vi "guangzi_16.vi"() -> ()   [LabVIEW 2016]
uses:
  <vilib>/Utility/file.llb/Write To Spreadsheet File (DBL).vi
panel:
  in  "采集开关":bool
  out "切片图":u32[](graph)
  in  "切片值":i32
  in  "选项卡控件":T1(tab)
  in  "对数":bool
  out "MCS8Dat Error":i32
  out "CHN Status":T2 {"Dummy" format="%.2f"; "Starts" format="%.2f"; "Sweeps" format="%.2f"; "Roirate" format="%.2f"; "RoiSum" format="%.2f"; "TotalSum" format="%.2f"; "Fifo full" format="%.2f"; "Runtime" format="%.2f"}
  out "Data":u32[](graph)
  out "Settings":T3 {"dummy3" format="%.2f"; "dummy2" format="%.2f"; "bitshift" format="%.0x"; "Active" format="%.0x"; "Offset" format="%.0x"; "Param" format="%.0x"; "dummy1" format="%.2f"; "Roipreset" format="%.2f"; "cftfak" format="%.0x"}
  out "通道数":i32
  out "Data 9":dbl[](graph)
  out "Data 2":u32[](graph)
  out "MCS8Dat Error 2":i32
  out "Settings 2":T3 {"dummy3" format="%.2f"; "dummy2" format="%.2f"; "bitshift" format="%.0x"; "Active" format="%.0x"; "Offset" format="%.0x"; "Param" format="%.0x"; "dummy1" format="%.2f"; "Roipreset" format="%.2f"; "cftfak" format="%.0x"}
  out "CHN Status 2":T2 {"Dummy" format="%.2f"; "Starts" format="%.2f"; "Sweeps" format="%.2f"; "Roirate" format="%.2f"; "RoiSum" format="%.2f"; "TotalSum" format="%.2f"; "Fifo full" format="%.2f"; "Runtime" format="%.2f"}
  out "通道数 2":i32
  in  "对数 2":bool
  out "Data10":dbl[](graph)
  out "Data 3":u32[](graph)
  out "MCS8Dat Error 3":i32
  out "Settings 3":T3 {"dummy3" format="%.2f"; "dummy2" format="%.2f"; "bitshift" format="%.0x"; "Active" format="%.0x"; "Offset" format="%.0x"; "Param" format="%.0x"; "dummy1" format="%.2f"; "Roipreset" format="%.2f"; "cftfak" format="%.0x"}
  out "CHN Status 3":T2 {"Dummy" format="%.2f"; "Starts" format="%.2f"; "Sweeps" format="%.2f"; "Roirate" format="%.2f"; "RoiSum" format="%.2f"; "TotalSum" format="%.2f"; "Fifo full" format="%.2f"; "Runtime" format="%.2f"}
  out "通道数 3":i32
  in  "对数 3":bool
  out "Data10 2":dbl[](graph)
  out "Data 4":u32[](graph)
  out "MCS8Dat Error 4":i32
  out "Settings 4":T3 {"dummy3" format="%.2f"; "dummy2" format="%.2f"; "bitshift" format="%.0x"; "Active" format="%.0x"; "Offset" format="%.0x"; "Param" format="%.0x"; "dummy1" format="%.2f"; "Roipreset" format="%.2f"; "cftfak" format="%.0x"}
  out "CHN Status 4":T2 {"Dummy" format="%.2f"; "Starts" format="%.2f"; "Sweeps" format="%.2f"; "Roirate" format="%.2f"; "RoiSum" format="%.2f"; "TotalSum" format="%.2f"; "Fifo full" format="%.2f"; "Runtime" format="%.2f"}
  out "通道数 4":i32
  in  "对数 4":bool
  out "Data10 3":dbl[](graph)
  out "Data 5":u32[](graph)
  out "MCS8Dat Error 5":i32
  out "Settings 5":T3 {"dummy3" format="%.2f"; "dummy2" format="%.2f"; "bitshift" format="%.0x"; "Active" format="%.0x"; "Offset" format="%.0x"; "Param" format="%.0x"; "dummy1" format="%.2f"; "Roipreset" format="%.2f"; "cftfak" format="%.0x"}
  out "CHN Status 5":T2 {"Dummy" format="%.2f"; "Starts" format="%.2f"; "Sweeps" format="%.2f"; "Roirate" format="%.2f"; "RoiSum" format="%.2f"; "TotalSum" format="%.2f"; "Fifo full" format="%.2f"; "Runtime" format="%.2f"}
  out "通道数 5":i32
  in  "对数 5":bool
  out "Data10 4":dbl[](graph)
  out "Data 6":u32[](graph)
  out "MCS8Dat Error 6":i32
  out "Settings 6":T3 {"dummy3" format="%.2f"; "dummy2" format="%.2f"; "bitshift" format="%.0x"; "Active" format="%.0x"; "Offset" format="%.0x"; "Param" format="%.0x"; "dummy1" format="%.2f"; "Roipreset" format="%.2f"; "cftfak" format="%.0x"}
  out "CHN Status 6":T2 {"Dummy" format="%.2f"; "Starts" format="%.2f"; "Sweeps" format="%.2f"; "Roirate" format="%.2f"; "RoiSum" format="%.2f"; "TotalSum" format="%.2f"; "Fifo full" format="%.2f"; "Runtime" format="%.2f"}
  out "通道数 6":i32
  in  "对数 6":bool
  out "Data10 5":dbl[](graph)
  out "Data 7":u32[](graph)
  out "MCS8Dat Error 7":i32
  out "Settings 7":T3 {"dummy3" format="%.2f"; "dummy2" format="%.2f"; "bitshift" format="%.0x"; "Active" format="%.0x"; "Offset" format="%.0x"; "Param" format="%.0x"; "dummy1" format="%.2f"; "Roipreset" format="%.2f"; "cftfak" format="%.0x"}
  out "CHN Status 7":T2 {"Dummy" format="%.2f"; "Starts" format="%.2f"; "Sweeps" format="%.2f"; "Roirate" format="%.2f"; "RoiSum" format="%.2f"; "TotalSum" format="%.2f"; "Fifo full" format="%.2f"; "Runtime" format="%.2f"}
  out "通道数 7":i32
  in  "对数 7":bool
  out "Data10 6":dbl[](graph)
  out "Data 8":u32[](graph)
  out "MCS8Dat Error 8":i32
  out "Settings 8":T3 {"dummy3" format="%.2f"; "dummy2" format="%.2f"; "bitshift" format="%.0x"; "Active" format="%.0x"; "Offset" format="%.0x"; "Param" format="%.0x"; "dummy1" format="%.2f"; "Roipreset" format="%.2f"; "cftfak" format="%.0x"}
  out "CHN Status 8":T2 {"Dummy" format="%.2f"; "Starts" format="%.2f"; "Sweeps" format="%.2f"; "Roirate" format="%.2f"; "RoiSum" format="%.2f"; "TotalSum" format="%.2f"; "Fifo full" format="%.2f"; "Runtime" format="%.2f"}
  out "通道数 8":i32
  in  "对数 8":bool
  out "Data10 7":dbl[](graph)
  out "Data9":u32[](graph)
  out "MCS8Dat Error 9":i32
  out "Settings 9":T3 {"dummy3" format="%.2f"; "dummy2" format="%.2f"; "bitshift" format="%.0x"; "Active" format="%.0x"; "Offset" format="%.0x"; "Param" format="%.0x"; "dummy1" format="%.2f"; "Roipreset" format="%.2f"; "cftfak" format="%.0x"}
  out "CHN Status 9":T2 {"Dummy" format="%.2f"; "Starts" format="%.2f"; "Sweeps" format="%.2f"; "Roirate" format="%.2f"; "RoiSum" format="%.2f"; "TotalSum" format="%.2f"; "Fifo full" format="%.2f"; "Runtime" format="%.2f"}
  out "通道数 9":i32
  in  "对数 9":bool
  out "Data108":dbl[](graph)
  in  "对数 10":bool
  out "通道数 10":i32
  out "CHN Status 10":T2 {"Dummy" format="%.2f"; "Starts" format="%.2f"; "Sweeps" format="%.2f"; "Roirate" format="%.2f"; "RoiSum" format="%.2f"; "TotalSum" format="%.2f"; "Fifo full" format="%.2f"; "Runtime" format="%.2f"}
  out "Settings 10":T3 {"dummy3" format="%.2f"; "dummy2" format="%.2f"; "bitshift" format="%.0x"; "Active" format="%.0x"; "Offset" format="%.0x"; "Param" format="%.0x"; "dummy1" format="%.2f"; "Roipreset" format="%.2f"; "cftfak" format="%.0x"}
  out "MCS8Dat Error 10":i32
  out "Data10 8":u32[](graph)
  out "Data10 9":dbl[](graph)
  in  "对数 11":bool
  out "通道数 11":i32
  out "CHN Status 11":T2 {"Dummy" format="%.2f"; "Starts" format="%.2f"; "Sweeps" format="%.2f"; "Roirate" format="%.2f"; "RoiSum" format="%.2f"; "TotalSum" format="%.2f"; "Fifo full" format="%.2f"; "Runtime" format="%.2f"}
  out "Settings 11":T3 {"dummy3" format="%.2f"; "dummy2" format="%.2f"; "bitshift" format="%.0x"; "Active" format="%.0x"; "Offset" format="%.0x"; "Param" format="%.0x"; "dummy1" format="%.2f"; "Roipreset" format="%.2f"; "cftfak" format="%.0x"}
  out "MCS8Dat Error 11":i32
  out "Data11":u32[](graph)
  out "Data10 10":dbl[](graph)
  in  "对数 12":bool
  out "通道数 12":i32
  out "CHN Status 12":T2 {"Dummy" format="%.2f"; "Starts" format="%.2f"; "Sweeps" format="%.2f"; "Roirate" format="%.2f"; "RoiSum" format="%.2f"; "TotalSum" format="%.2f"; "Fifo full" format="%.2f"; "Runtime" format="%.2f"}
  out "Settings 12":T3 {"dummy3" format="%.2f"; "dummy2" format="%.2f"; "bitshift" format="%.0x"; "Active" format="%.0x"; "Offset" format="%.0x"; "Param" format="%.0x"; "dummy1" format="%.2f"; "Roipreset" format="%.2f"; "cftfak" format="%.0x"}
  out "MCS8Dat Error 12":i32
  out "Data12":u32[](graph)
  out "Data10 11":dbl[](graph)
  in  "对数 13":bool
  out "通道数 13":i32
  out "CHN Status 13":T2 {"Dummy" format="%.2f"; "Starts" format="%.2f"; "Sweeps" format="%.2f"; "Roirate" format="%.2f"; "RoiSum" format="%.2f"; "TotalSum" format="%.2f"; "Fifo full" format="%.2f"; "Runtime" format="%.2f"}
  out "Settings 13":T3 {"dummy3" format="%.2f"; "dummy2" format="%.2f"; "bitshift" format="%.0x"; "Active" format="%.0x"; "Offset" format="%.0x"; "Param" format="%.0x"; "dummy1" format="%.2f"; "Roipreset" format="%.2f"; "cftfak" format="%.0x"}
  out "MCS8Dat Error 13":i32
  out "Data13":u32[](graph)
  out "Data10 12":dbl[](graph)
  in  "对数 14":bool
  out "通道数 14":i32
  out "CHN Status 14":T2 {"Dummy" format="%.2f"; "Starts" format="%.2f"; "Sweeps" format="%.2f"; "Roirate" format="%.2f"; "RoiSum" format="%.2f"; "TotalSum" format="%.2f"; "Fifo full" format="%.2f"; "Runtime" format="%.2f"}
  out "Settings 14":T3 {"dummy3" format="%.2f"; "dummy2" format="%.2f"; "bitshift" format="%.0x"; "Active" format="%.0x"; "Offset" format="%.0x"; "Param" format="%.0x"; "dummy1" format="%.2f"; "Roipreset" format="%.2f"; "cftfak" format="%.0x"}
  out "MCS8Dat Error 14":i32
  out "Data14":u32[](graph)
  out "Data10 13":dbl[](graph)
  in  "对数 15":bool
  out "通道数 15":i32
  out "CHN Status 15":T2 {"Dummy" format="%.2f"; "Starts" format="%.2f"; "Sweeps" format="%.2f"; "Roirate" format="%.2f"; "RoiSum" format="%.2f"; "TotalSum" format="%.2f"; "Fifo full" format="%.2f"; "Runtime" format="%.2f"}
  out "Settings 15":T3 {"dummy3" format="%.2f"; "dummy2" format="%.2f"; "bitshift" format="%.0x"; "Active" format="%.0x"; "Offset" format="%.0x"; "Param" format="%.0x"; "dummy1" format="%.2f"; "Roipreset" format="%.2f"; "cftfak" format="%.0x"}
  out "MCS8Dat Error 15":i32
  out "Data15":u32[](graph)
  out "Data10 14":dbl[](graph)
  in  "对数 16":bool
  out "通道数 16":i32
  out "CHN Status 16":T2 {"Dummy" format="%.2f"; "Starts" format="%.2f"; "Sweeps" format="%.2f"; "Roirate" format="%.2f"; "RoiSum" format="%.2f"; "TotalSum" format="%.2f"; "Fifo full" format="%.2f"; "Runtime" format="%.2f"}
  out "Settings 16":T3 {"dummy3" format="%.2f"; "dummy2" format="%.2f"; "bitshift" format="%.0x"; "Active" format="%.0x"; "Offset" format="%.0x"; "Param" format="%.0x"; "dummy1" format="%.2f"; "Roipreset" format="%.2f"; "cftfak" format="%.0x"}
  out "MCS8Dat Error 16":i32
  out "Data16":u32[](graph)
  out "Data10 15":dbl[](graph)
  in  "子开关":bool
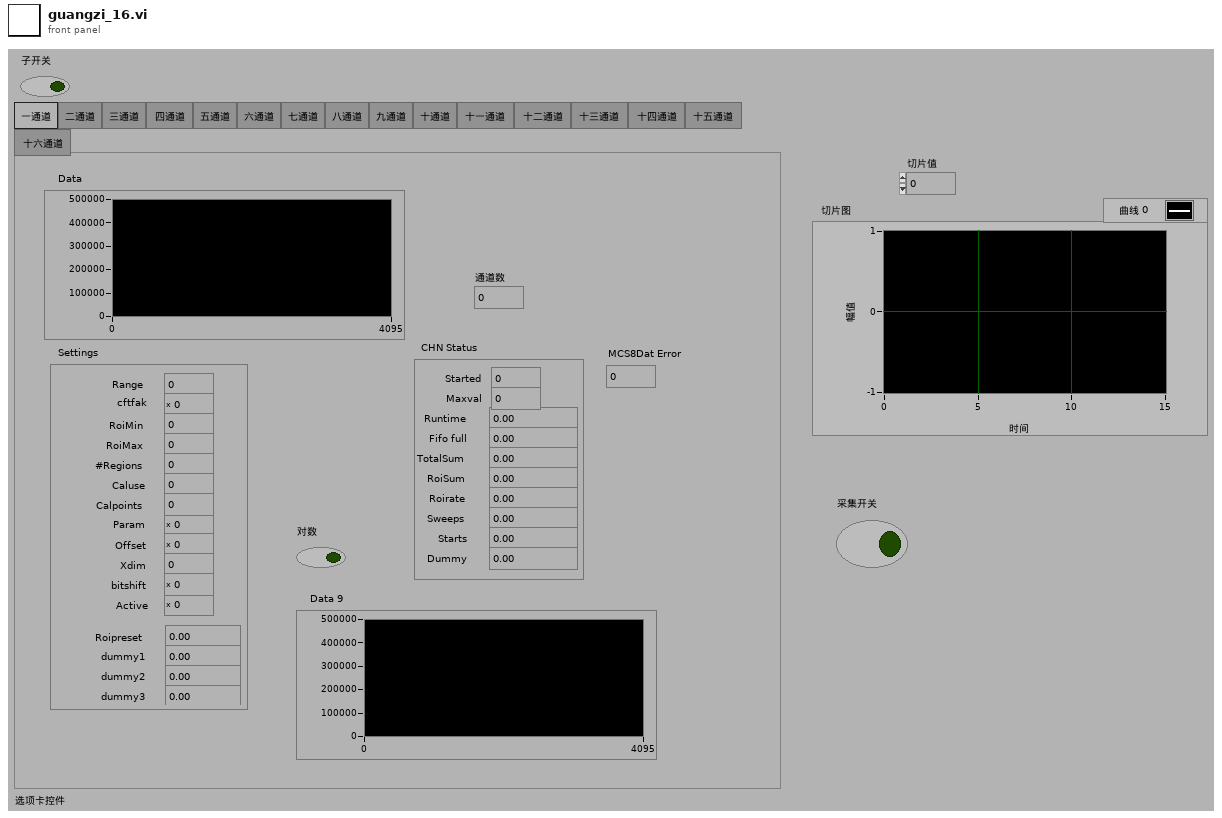
[diagram p1: front panel]
types:
  T1 = enum32{"一通道", "二通道", "三通道", "四通道 ", "五通道", "六通道", "七通道", "八通道", "九通道", "十通道", "十一通道 ", "十二通道 ", "十三通道 ", "十四通道 ", "十五通道 ", "十六通道 "}
  T2 = cluster{"Started":i32, "Maxval":u32, "Runtime":dbl, "Fifo full":dbl, "TotalSum":dbl, "RoiSum":dbl, "Roirate":dbl, "Sweeps":dbl, "Starts":dbl, "Dummy":dbl}
  T3 = cluster{"Range":i32, "cftfak":i32, "RoiMin":i32, "RoiMax":i32, "#Regions":i32, "Caluse":i32, "Calpoints":i32, "Param":i32, "Offset":i32, "Xdim":i32, "bitshift":i32, "Active":i32, "Roipreset":dbl, "dummy1":dbl, "dummy2":dbl, "dummy3":dbl}
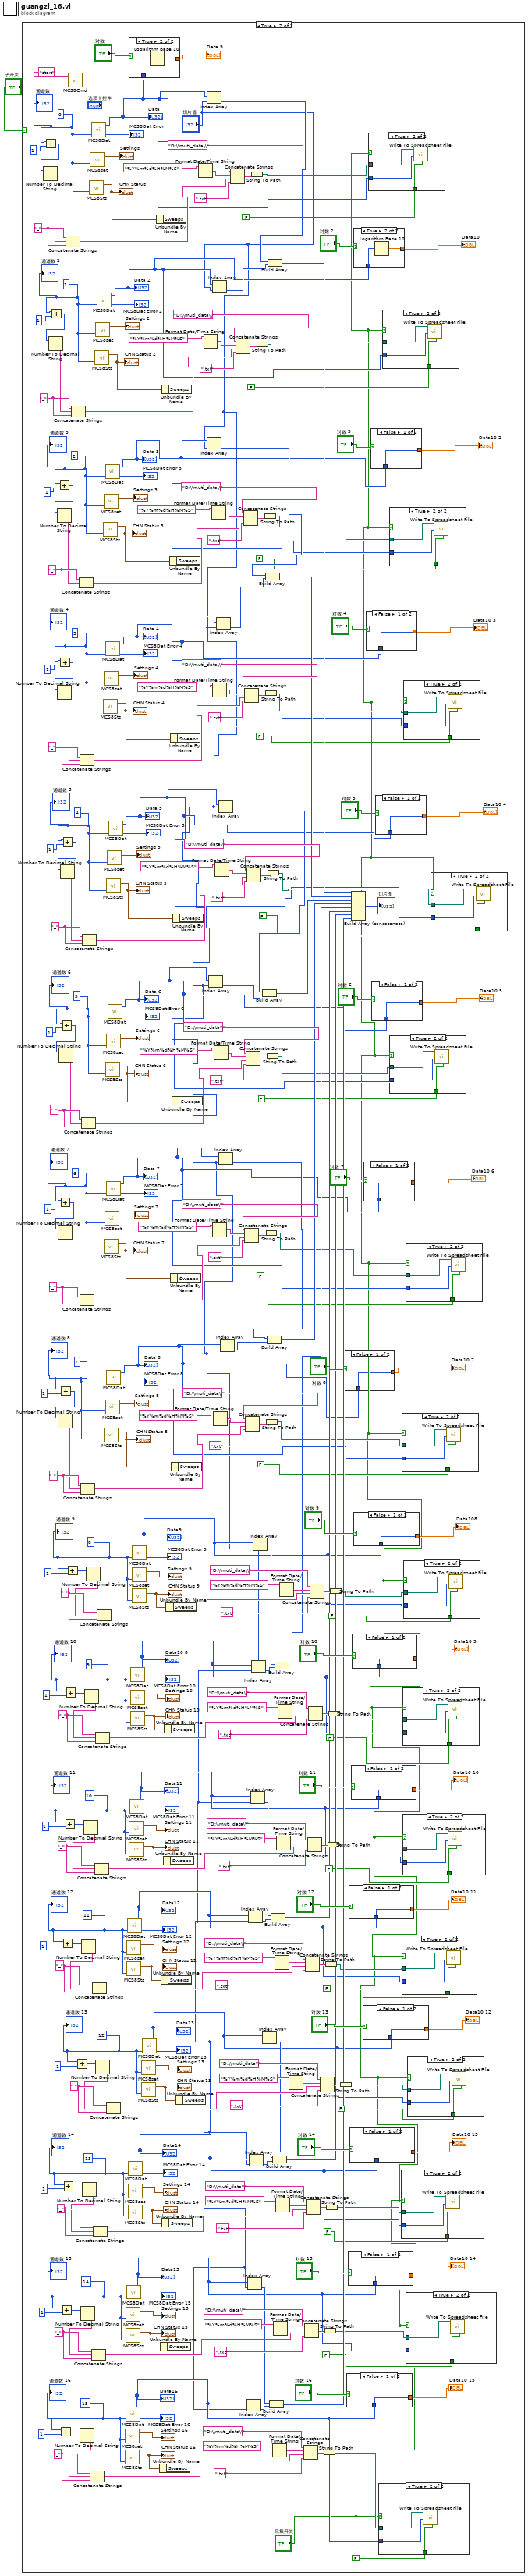
[diagram p0: block diagram]
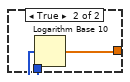
[diagram p19: hidden frame]
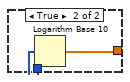
[diagram p20: hidden frame]
diagram:
  n1 = case shown="True" "子开关" {
    frame False {
    }
    frame True {
      w62 = "_"
      w68 = 15
      w78 = "_"
      w84 = 14
      w97 = "_"
      w103 = 13
      w113 = "_"
      w119 = 12
      w132 = "_"
      w138 = 11
      w148 = "_"
      w154 = 10
      w167 = "_"
      w173 = 9
      w183 = "_"
      w189 = 8
      w222 = 7
      w230 = "_"
      w236 = 6
      w244 = "_"
      w250 = 5
      w258 = "_"
      w264 = 4
      w272 = "_"
      w278 = 3
      w286 = "_"
      w292 = 2
      w300 = "_"
      w306 = 1
      w314 = "_"
      w319 = 0
      w327 = "_"
      n2 = Add(x=w319, y=1) -> (x+y=w322:i32)
      n3 = Number To Decimal String(number=w322) -> (decimal integer string=w326:string)  [unwired: 1 in]
      n4 = Add(x=w306, y=1) -> (x+y=w309:i32)
      n5 = Number To Decimal String(number=w309) -> (decimal integer string=w313:string)  [unwired: 1 in]
      n6 = Add(x=w292, y=1) -> (x+y=w295:i32)
      n7 = Number To Decimal String(number=w295) -> (decimal integer string=w299:string)  [unwired: 1 in]
      n8 = Add(x=w278, y=1) -> (x+y=w281:i32)
      n9 = Number To Decimal String(number=w281) -> (decimal integer string=w285:string)  [unwired: 1 in]
      n10 = Add(x=w236, y=1) -> (x+y=w239:i32)
      n11 = Number To Decimal String(number=w239) -> (decimal integer string=w243:string)  [unwired: 1 in]
      n12 = Add(x=w222, y=1) -> (x+y=w225:i32)
      n13 = Number To Decimal String(number=w225) -> (decimal integer string=w229:string)  [unwired: 1 in]
      n14 = Add(x=w68, y=1) -> (x+y=w69:i32)
      n15 = Add(x=w250, y=1) -> (x+y=w253:i32)
      n16 = Number To Decimal String(number=w253) -> (decimal integer string=w257:string)  [unwired: 1 in]
      n17 = Add(x=w84, y=1) -> (x+y=w85:i32)
      n18 = Add(x=w264, y=1) -> (x+y=w267:i32)
      n19 = Number To Decimal String(number=w267) -> (decimal integer string=w271:string)  [unwired: 1 in]
      n20 = Add(x=w138, y=1) -> (x+y=w139:i32)
      n21 = Add(x=w103, y=1) -> (x+y=w104:i32)
      n22 = Add(x=w154, y=1) -> (x+y=w155:i32)
      n23 = Add(x=w173, y=1) -> (x+y=w174:i32)
      n24 = Concatenate Strings(w327, w326, w327) -> (w325:string)
      n25 = Add(x=w189, y=1) -> (x+y=w190:i32)
      n26 = call "MCS8Cmd.vi"("Command"="start") -> ()  [unwired: 2 in, 1 out]
      n27 = Concatenate Strings(w314, w313, w314) -> (w312:string)
      n28 = Add(x=w119, y=1) -> (x+y=w120:i32)
      n29 = Concatenate Strings(w300, w299, w300) -> (w298:string)
      n30 = Concatenate Strings(w286, w285, w286) -> (w284:string)
      n31 = Number To Decimal String(number=w69) -> (decimal integer string=w61:string)  [unwired: 1 in]
      n32 = Concatenate Strings(w244, w243, w244) -> (w242:string)
      n33 = Concatenate Strings(w230, w229, w230) -> (w228:string)
      n34 = Number To Decimal String(number=w85) -> (decimal integer string=w77:string)  [unwired: 1 in]
      n35 = Concatenate Strings(w258, w257, w258) -> (w256:string)
      n36 = Number To Decimal String(number=w139) -> (decimal integer string=w131:string)  [unwired: 1 in]
      n37 = Concatenate Strings(w272, w271, w272) -> (w270:string)
      n38 = Number To Decimal String(number=w104) -> (decimal integer string=w96:string)  [unwired: 1 in]
      n39 = Number To Decimal String(number=w155) -> (decimal integer string=w147:string)  [unwired: 1 in]
      n40 = Number To Decimal String(number=w174) -> (decimal integer string=w166:string)  [unwired: 1 in]
      n41 = Number To Decimal String(number=w190) -> (decimal integer string=w182:string)  [unwired: 1 in]
      n42 = call "MCS8Sts.vi"("CHN #"=w319) -> ("CHN Status"=w332:T2)  [unwired: 1 in, 1 out]
      "CHN Status" <- w332
      n43 = call "MCS8set.vi"("Spect #"=w319) -> ("Settings"=→"Settings":T3)  [unwired: 1 in, 1 out]
      n44 = Concatenate Strings(w62, w61, w62) -> (w57:string)
      n45 = Concatenate Strings(w78, w77, w78) -> (w73:string)
      n46 = call "MCS8Dat.vi"("Spectrum #"=w319) -> ("MCS8Dat Error"=→"MCS8Dat Error":i32, "Data"=w5:u32[])  [unwired: 2 in, 1 out]
      "Data" <- w5
      n47 = Concatenate Strings(w132, w131, w132) -> (w127:string)
      n48 = Concatenate Strings(w97, w96, w97) -> (w92:string)
      n49 = Concatenate Strings(w148, w147, w148) -> (w143:string)
      n50 = call "MCS8Sts.vi"("CHN #"=w306) -> ("CHN Status"=w192:T2)  [unwired: 1 in, 1 out]
      "CHN Status 2" <- w192
      n51 = Concatenate Strings(w167, w166, w167) -> (w162:string)
      n52 = call "MCS8set.vi"("Spect #"=w306) -> ("Settings"=→"Settings 2":T3)  [unwired: 1 in, 1 out]
      n53 = Number To Decimal String(number=w120) -> (decimal integer string=w112:string)  [unwired: 1 in]
      n54 = call "MCS8Dat.vi"("Spectrum #"=w306) -> ("MCS8Dat Error"=→"MCS8Dat Error 2":i32, "Data"=w8:u32[])  [unwired: 2 in, 1 out]
      "Data 2" <- w8
      n55 = Concatenate Strings(w183, w182, w183) -> (w178:string)
      n56 = call "MCS8Sts.vi"("CHN #"=w292) -> ("CHN Status"=w305:T2)  [unwired: 1 in, 1 out]
      "CHN Status 3" <- w305
      n57 = call "MCS8Sts.vi"("CHN #"=w278) -> ("CHN Status"=w291:T2)  [unwired: 1 in, 1 out]
      "CHN Status 4" <- w291
      n58 = call "MCS8set.vi"("Spect #"=w292) -> ("Settings"=→"Settings 3":T3)  [unwired: 1 in, 1 out]
      n59 = call "MCS8Sts.vi"("CHN #"=w236) -> ("CHN Status"=w249:T2)  [unwired: 1 in, 1 out]
      "CHN Status 7" <- w249
      n60 = call "MCS8set.vi"("Spect #"=w278) -> ("Settings"=→"Settings 4":T3)  [unwired: 1 in, 1 out]
      n61 = call "MCS8Sts.vi"("CHN #"=w222) -> ("CHN Status"=w235:T2)  [unwired: 1 in, 1 out]
      "CHN Status 8" <- w235
      n62 = call "MCS8set.vi"("Spect #"=w236) -> ("Settings"=→"Settings 7":T3)  [unwired: 1 in, 1 out]
      n63 = call "MCS8Dat.vi"("Spectrum #"=w292) -> ("MCS8Dat Error"=→"MCS8Dat Error 3":i32, "Data"=w11:u32[])  [unwired: 2 in, 1 out]
      "Data 3" <- w11
      n64 = call "MCS8Sts.vi"("CHN #"=w250) -> ("CHN Status"=w263:T2)  [unwired: 1 in, 1 out]
      "CHN Status 6" <- w263
      n65 = call "MCS8set.vi"("Spect #"=w222) -> ("Settings"=→"Settings 8":T3)  [unwired: 1 in, 1 out]
      n66 = call "MCS8Dat.vi"("Spectrum #"=w278) -> ("MCS8Dat Error"=→"MCS8Dat Error 4":i32, "Data"=w14:u32[])  [unwired: 2 in, 1 out]
      "Data 4" <- w14
      n67 = call "MCS8Sts.vi"("CHN #"=w264) -> ("CHN Status"=w277:T2)  [unwired: 1 in, 1 out]
      "CHN Status 5" <- w277
      n68 = call "MCS8set.vi"("Spect #"=w250) -> ("Settings"=→"Settings 6":T3)  [unwired: 1 in, 1 out]
      n69 = call "MCS8Dat.vi"("Spectrum #"=w236) -> ("MCS8Dat Error"=→"MCS8Dat Error 7":i32, "Data"=w23:u32[])  [unwired: 2 in, 1 out]
      "Data 7" <- w23
      n70 = call "MCS8Dat.vi"("Spectrum #"=w222) -> ("MCS8Dat Error"=→"MCS8Dat Error 8":i32, "Data"=w26:u32[])  [unwired: 2 in, 1 out]
      "Data 8" <- w26
      n71 = Concatenate Strings(w113, w112, w113) -> (w108:string)
      n72 = call "MCS8set.vi"("Spect #"=w264) -> ("Settings"=→"Settings 5":T3)  [unwired: 1 in, 1 out]
      n73 = call "MCS8Dat.vi"("Spectrum #"=w250) -> ("MCS8Dat Error"=→"MCS8Dat Error 6":i32, "Data"=w20:u32[])  [unwired: 2 in, 1 out]
      "Data 6" <- w20
      n74 = call "MCS8Dat.vi"("Spectrum #"=w264) -> ("MCS8Dat Error"=→"MCS8Dat Error 5":i32, "Data"=w17:u32[])  [unwired: 2 in, 1 out]
      "Data 5" <- w17
      n75 = call "MCS8set.vi"("Spect #"=w68) -> ("Settings"=→"Settings 16":T3)  [unwired: 1 in, 1 out]
      n76 = call "MCS8Sts.vi"("CHN #"=w68) -> ("CHN Status"=w63:T2)  [unwired: 1 in, 1 out]
      "CHN Status 16" <- w63
      n77 = call "MCS8Dat.vi"("Spectrum #"=w68) -> ("MCS8Dat Error"=→"MCS8Dat Error 16":i32, "Data"=w50:u32[])  [unwired: 2 in, 1 out]
      "Data16" <- w50
      n78 = call "MCS8set.vi"("Spect #"=w84) -> ("Settings"=→"Settings 15":T3)  [unwired: 1 in, 1 out]
      n79 = call "MCS8Sts.vi"("CHN #"=w84) -> ("CHN Status"=w79:T2)  [unwired: 1 in, 1 out]
      "CHN Status 15" <- w79
      n80 = call "MCS8Dat.vi"("Spectrum #"=w84) -> ("MCS8Dat Error"=→"MCS8Dat Error 15":i32, "Data"=w47:u32[])  [unwired: 2 in, 1 out]
      "Data15" <- w47
      n81 = call "MCS8set.vi"("Spect #"=w138) -> ("Settings"=→"Settings 12":T3)  [unwired: 1 in, 1 out]
      n82 = call "MCS8Sts.vi"("CHN #"=w138) -> ("CHN Status"=w133:T2)  [unwired: 1 in, 1 out]
      "CHN Status 12" <- w133
      n83 = call "MCS8Dat.vi"("Spectrum #"=w138) -> ("MCS8Dat Error"=→"MCS8Dat Error 12":i32, "Data"=w38:u32[])  [unwired: 2 in, 1 out]
      "Data12" <- w38
      n84 = call "MCS8set.vi"("Spect #"=w103) -> ("Settings"=→"Settings 14":T3)  [unwired: 1 in, 1 out]
      n85 = call "MCS8Sts.vi"("CHN #"=w103) -> ("CHN Status"=w98:T2)  [unwired: 1 in, 1 out]
      "CHN Status 14" <- w98
      n86 = call "MCS8Dat.vi"("Spectrum #"=w103) -> ("MCS8Dat Error"=→"MCS8Dat Error 14":i32, "Data"=w44:u32[])  [unwired: 2 in, 1 out]
      "Data14" <- w44
      n87 = case shown="True" "对数" {
        tunnel: w5 -> [w427 w428]
        tunnel: [w427 w429] -> w207
        frame False {
        }
        frame True {
          n88 = Logarithm Base 10(1:w428) -> (0:w429:dbl[])
        }
      }
      "Data 9" <- w207
      n89 = call "MCS8set.vi"("Spect #"=w154) -> ("Settings"=→"Settings 11":T3)  [unwired: 1 in, 1 out]
      n90 = call "MCS8Sts.vi"("CHN #"=w154) -> ("CHN Status"=w149:T2)  [unwired: 1 in, 1 out]
      "CHN Status 11" <- w149
      n91 = call "MCS8Dat.vi"("Spectrum #"=w154) -> ("MCS8Dat Error"=→"MCS8Dat Error 11":i32, "Data"=w35:u32[])  [unwired: 2 in, 1 out]
      "Data11" <- w35
      n92 = call "MCS8set.vi"("Spect #"=w173) -> ("Settings"=→"Settings 10":T3)  [unwired: 1 in, 1 out]
      n93 = call "MCS8Sts.vi"("CHN #"=w173) -> ("CHN Status"=w168:T2)  [unwired: 1 in, 1 out]
      "CHN Status 10" <- w168
      n94 = call "MCS8Dat.vi"("Spectrum #"=w173) -> ("MCS8Dat Error"=→"MCS8Dat Error 10":i32, "Data"=w32:u32[])  [unwired: 2 in, 1 out]
      "Data10 8" <- w32
      n95 = call "MCS8set.vi"("Spect #"=w189) -> ("Settings"=→"Settings 9":T3)  [unwired: 1 in, 1 out]
      n96 = call "MCS8Sts.vi"("CHN #"=w189) -> ("CHN Status"=w184:T2)  [unwired: 1 in, 1 out]
      "CHN Status 9" <- w184
      n97 = call "MCS8Dat.vi"("Spectrum #"=w189) -> ("MCS8Dat Error"=→"MCS8Dat Error 9":i32, "Data"=w29:u32[])  [unwired: 2 in, 1 out]
      "Data9" <- w29
      n98 = call "MCS8set.vi"("Spect #"=w119) -> ("Settings"=→"Settings 13":T3)  [unwired: 1 in, 1 out]
      n99 = call "MCS8Sts.vi"("CHN #"=w119) -> ("CHN Status"=w114:T2)  [unwired: 1 in, 1 out]
      "CHN Status 13" <- w114
      n100 = call "MCS8Dat.vi"("Spectrum #"=w119) -> ("MCS8Dat Error"=→"MCS8Dat Error 13":i32, "Data"=w41:u32[])  [unwired: 2 in, 1 out]
      "Data13" <- w41
      n101 = Unbundle By Name(w332) -> ()  [unwired: 1 out]
      n102 = Unbundle By Name(w63) -> ()  [unwired: 1 out]
      n103 = Unbundle By Name(w79) -> ()  [unwired: 1 out]
      n104 = Unbundle By Name(w133) -> ()  [unwired: 1 out]
      n105 = Unbundle By Name(w192) -> ()  [unwired: 1 out]
      n106 = Unbundle By Name(w98) -> ()  [unwired: 1 out]
      n107 = Unbundle By Name(w149) -> ()  [unwired: 1 out]
      n108 = Unbundle By Name(w168) -> ()  [unwired: 1 out]
      n109 = Unbundle By Name(w184) -> ()  [unwired: 1 out]
      n110 = Unbundle By Name(w305) -> ()  [unwired: 1 out]
      n111 = Unbundle By Name(w291) -> ()  [unwired: 1 out]
      n112 = Unbundle By Name(w249) -> ()  [unwired: 1 out]
      n113 = Unbundle By Name(w235) -> ()  [unwired: 1 out]
      n114 = Unbundle By Name(w263) -> ()  [unwired: 1 out]
      n115 = Unbundle By Name(w277) -> ()  [unwired: 1 out]
      n116 = Unbundle By Name(w114) -> ()  [unwired: 1 out]
      n117 = Format Date/Time String(time format string (%c)="%Y%m%d%H%M%S") -> (date/time string=w323:string)  [unwired: 2 in]
      n118 = Format Date/Time String(time format string (%c)="%Y%m%d%H%M%S") -> (date/time string=w310:string)  [unwired: 2 in]
      n119 = Index Array(array=w5, index="切片值") -> (element=w215:u32)
      n120 = Index Array(array=w11, index="切片值") -> (element=w217:u32)
      n121 = Index Array(array=w20, index="切片值") -> (element=w219:u32)
      n122 = Format Date/Time String(time format string (%c)="%Y%m%d%H%M%S") -> (date/time string=w296:string)  [unwired: 2 in]
      n123 = Index Array(array=w8, index="切片值") -> (element=w214:u32)
      n124 = Format Date/Time String(time format string (%c)="%Y%m%d%H%M%S") -> (date/time string=w282:string)  [unwired: 2 in]
      n125 = Format Date/Time String(time format string (%c)="%Y%m%d%H%M%S") -> (date/time string=w240:string)  [unwired: 2 in]
      n126 = Format Date/Time String(time format string (%c)="%Y%m%d%H%M%S") -> (date/time string=w226:string)  [unwired: 2 in]
      n127 = Format Date/Time String(time format string (%c)="%Y%m%d%H%M%S") -> (date/time string=w254:string)  [unwired: 2 in]
      n128 = Format Date/Time String(time format string (%c)="%Y%m%d%H%M%S") -> (date/time string=w268:string)  [unwired: 2 in]
      n129 = Index Array(array=w14, index="切片值") -> (element=w216:u32)
      n130 = Index Array(array=w23, index="切片值") -> (element=w220:u32)
      n131 = Index Array(array=w17, index="切片值") -> (element=w218:u32)
      n132 = Index Array(array=w26, index="切片值") -> (element=w221:u32)
      n133 = Concatenate Strings("D:\\muti_data\\", w323, w325, ".txt") -> (w329:string)
      n134 = Concatenate Strings("D:\\muti_data\\", w310, w312, ".txt") -> (w316:string)
      n135 = Concatenate Strings("D:\\muti_data\\", w296, w298, ".txt") -> (w302:string)
      n136 = Concatenate Strings("D:\\muti_data\\", w282, w284, ".txt") -> (w288:string)
      n137 = Concatenate Strings("D:\\muti_data\\", w240, w242, ".txt") -> (w246:string)
      n138 = Concatenate Strings("D:\\muti_data\\", w226, w228, ".txt") -> (w232:string)
      n139 = Concatenate Strings("D:\\muti_data\\", w254, w256, ".txt") -> (w260:string)
      n140 = Index Array(array=w50, index="切片值") -> (element=w54:u32)
      n141 = Concatenate Strings("D:\\muti_data\\", w268, w270, ".txt") -> (w274:string)
      n142 = Index Array(array=w47, index="切片值") -> (element=w53:u32)
      n143 = Index Array(array=w38, index="切片值") -> (element=w123:u32)
      n144 = Index Array(array=w44, index="切片值") -> (element=w88:u32)
      n145 = String To Path(string=w329) -> (path=w6:path)
      n146 = Index Array(array=w35, index="切片值") -> (element=w124:u32)
      n147 = Index Array(array=w32, index="切片值") -> (element=w158:u32)
      n148 = Index Array(array=w29, index="切片值") -> (element=w159:u32)
      n149 = String To Path(string=w316) -> (path=w9:path)
      n150 = Build Array(w218, w219) -> (w211:u32[])
      n151 = Index Array(array=w41, index="切片值") -> (element=w89:u32)
      n152 = String To Path(string=w302) -> (path=w12:path)
      n153 = String To Path(string=w288) -> (path=w15:path)
      n154 = String To Path(string=w246) -> (path=w24:path)
      n155 = String To Path(string=w232) -> (path=w27:path)
      n156 = Build Array(w217, w216) -> (w212:u32[])
      n157 = String To Path(string=w260) -> (path=w21:path)
      n158 = String To Path(string=w274) -> (path=w18:path)
      n159 = Build Array(w220, w221) -> (w210:u32[])
      n160 = Build Array(w215, w214) -> (w213:u32[])
      n161 = Build Array(w53, w54) -> (w52:u32[])
      n162 = Build Array(w124, w123) -> (w122:u32[])
      n163 = Build Array(w89, w88) -> (w87:u32[])
      n164 = Format Date/Time String(time format string (%c)="%Y%m%d%H%M%S") -> (date/time string=w59:string)  [unwired: 2 in]
      n165 = Format Date/Time String(time format string (%c)="%Y%m%d%H%M%S") -> (date/time string=w75:string)  [unwired: 2 in]
      n166 = Build Array(w159, w158) -> (w157:u32[])
      n167 = Format Date/Time String(time format string (%c)="%Y%m%d%H%M%S") -> (date/time string=w129:string)  [unwired: 2 in]
      n168 = Format Date/Time String(time format string (%c)="%Y%m%d%H%M%S") -> (date/time string=w94:string)  [unwired: 2 in]
      n169 = Format Date/Time String(time format string (%c)="%Y%m%d%H%M%S") -> (date/time string=w145:string)  [unwired: 2 in]
      n170 = Format Date/Time String(time format string (%c)="%Y%m%d%H%M%S") -> (date/time string=w164:string)  [unwired: 2 in]
      n171 = Format Date/Time String(time format string (%c)="%Y%m%d%H%M%S") -> (date/time string=w180:string)  [unwired: 2 in]
      n172 = Format Date/Time String(time format string (%c)="%Y%m%d%H%M%S") -> (date/time string=w110:string)  [unwired: 2 in]
      n173 = Concatenate Strings("D:\\muti_data\\", w59, w57, ".txt") -> (w55:string)
      n174 = Concatenate Strings("D:\\muti_data\\", w75, w73, ".txt") -> (w71:string)
      n175 = Concatenate Strings("D:\\muti_data\\", w129, w127, ".txt") -> (w125:string)
      n176 = Concatenate Strings("D:\\muti_data\\", w94, w92, ".txt") -> (w90:string)
      n177 = Concatenate Strings("D:\\muti_data\\", w145, w143, ".txt") -> (w141:string)
      n178 = Concatenate Strings("D:\\muti_data\\", w164, w162, ".txt") -> (w160:string)
      n179 = Concatenate Strings("D:\\muti_data\\", w180, w178, ".txt") -> (w176:string)
      n180 = Concatenate Strings("D:\\muti_data\\", w110, w108, ".txt") -> (w106:string)
      n181 = String To Path(string=w55) -> (path=w51:path)
      n182 = String To Path(string=w71) -> (path=w48:path)
      n183 = String To Path(string=w125) -> (path=w39:path)
      n184 = String To Path(string=w90) -> (path=w43:path)
      n185 = String To Path(string=w141) -> (path=w36:path)
      n186 = String To Path(string=w160) -> (path=w33:path)
      n187 = String To Path(string=w176) -> (path=w30:path)
      n188 = String To Path(string=w106) -> (path=w42:path)
      n189 = case shown="False" "对数 8" {
        tunnel: w26 -> [w406 w408]
        tunnel: [w406 w407] -> w193
        frame False {
        }
        frame True {
          n190 = Logarithm Base 10(1:w408) -> (0:w407:dbl[])
        }
      }
      "Data10 7" <- w193
      n191 = case shown="False" "对数 16" {
        tunnel: w50 -> [w382 w384]
        tunnel: [w382 w383] -> w64
        frame False {
        }
        frame True {
          n192 = Logarithm Base 10(1:w384) -> (0:w383:dbl[])
        }
      }
      "Data10 15" <- w64
      n193 = case shown="False" "对数 15" {
        tunnel: w47 -> [w385 w387]
        tunnel: [w385 w386] -> w80
        frame False {
        }
        frame True {
          n194 = Logarithm Base 10(1:w387) -> (0:w386:dbl[])
        }
      }
      "Data10 14" <- w80
      n195 = case shown="False" "对数 12" {
        tunnel: w38 -> [w394 w396]
        tunnel: [w394 w395] -> w134
        frame False {
        }
        frame True {
          n196 = Logarithm Base 10(1:w396) -> (0:w395:dbl[])
        }
      }
      "Data10 11" <- w134
      n197 = case shown="False" "对数 14" {
        tunnel: w44 -> [w388 w390]
        tunnel: [w388 w389] -> w99
        frame False {
        }
        frame True {
          n198 = Logarithm Base 10(1:w390) -> (0:w389:dbl[])
        }
      }
      "Data10 13" <- w99
      n199 = case shown="False" "对数 11" {
        tunnel: w35 -> [w397 w399]
        tunnel: [w397 w398] -> w150
        frame False {
        }
        frame True {
          n200 = Logarithm Base 10(1:w399) -> (0:w398:dbl[])
        }
      }
      "Data10 10" <- w150
      n201 = Build Array (concatenate)(w213, w212, w211, w210, w157, w122, w87, w52) -> (→"切片图":u32[])
      n202 = case shown="False" "对数 10" {
        tunnel: w32 -> [w400 w402]
        tunnel: [w400 w401] -> w169
        frame False {
        }
        frame True {
          n203 = Logarithm Base 10(1:w402) -> (0:w401:dbl[])
        }
      }
      "Data10 9" <- w169
      n204 = case shown="True" "对数 2" {
        tunnel: w8 -> [w424 w426]
        tunnel: [w424 w425] -> w205
        frame False {
        }
        frame True {
          n205 = Logarithm Base 10(1:w426) -> (0:w425:dbl[])
        }
      }
      "Data10" <- w205
      n206 = case shown="False" "对数 9" {
        tunnel: w29 -> [w403 w405]
        tunnel: [w403 w404] -> w185
        frame False {
        }
        frame True {
          n207 = Logarithm Base 10(1:w405) -> (0:w404:dbl[])
        }
      }
      "Data108" <- w185
      n208 = case shown="False" "对数 13" {
        tunnel: w41 -> [w391 w393]
        tunnel: [w391 w392] -> w115
        frame False {
        }
        frame True {
          n209 = Logarithm Base 10(1:w393) -> (0:w392:dbl[])
        }
      }
      "Data10 12" <- w115
      n210 = case shown="False" "对数 7" {
        tunnel: w23 -> [w409 w411]
        tunnel: [w409 w410] -> w195
        frame False {
        }
        frame True {
          n211 = Logarithm Base 10(1:w411) -> (0:w410:dbl[])
        }
      }
      "Data10 6" <- w195
      n212 = case shown="False" "对数 4" {
        tunnel: w14 -> [w418 w420]
        tunnel: [w418 w419] -> w201
        frame False {
        }
        frame True {
          n213 = Logarithm Base 10(1:w420) -> (0:w419:dbl[])
        }
      }
      "Data10 3" <- w201
      n214 = case shown="True" "采集开关" {
        tunnel: w6 -> [_ w336]
        tunnel: w5 -> [_ w335]
        tunnel: FALSE -> [_ w334]
        frame False {
        }
        frame True {
          n215 = call-poly <vilib>:"Write To Spreadsheet File.vi"("transpose? (no:F)"=w334, "1D data"=w335, "file path (dialog if empty)"=w336) -> ()  [unwired: 5 in, 1 out]
        }
      }
      n216 = case shown="False" "对数 3" {
        tunnel: w11 -> [w421 w423]
        tunnel: [w421 w422] -> w203
        frame False {
        }
        frame True {
          n217 = Logarithm Base 10(1:w423) -> (0:w422:dbl[])
        }
      }
      "Data10 2" <- w203
      n218 = case shown="False" "对数 6" {
        tunnel: w20 -> [w412 w414]
        tunnel: [w412 w413] -> w197
        frame False {
        }
        frame True {
          n219 = Logarithm Base 10(1:w414) -> (0:w413:dbl[])
        }
      }
      "Data10 5" <- w197
      n220 = case shown="False" "对数 5" {
        tunnel: w17 -> [w415 w417]
        tunnel: [w415 w416] -> w199
        frame False {
        }
        frame True {
          n221 = Logarithm Base 10(1:w417) -> (0:w416:dbl[])
        }
      }
      "Data10 4" <- w199
      n222 = case shown="True" "采集开关" {
        tunnel: w51 -> [_ w381]
        tunnel: w50 -> [_ w380]
        tunnel: FALSE -> [_ w379]
        frame False {
        }
        frame True {
          n223 = call-poly <vilib>:"Write To Spreadsheet File.vi"("transpose? (no:F)"=w379, "1D data"=w380, "file path (dialog if empty)"=w381) -> ()  [unwired: 5 in, 1 out]
        }
      }
      n224 = case shown="True" "采集开关" {
        tunnel: w9 -> [_ w339]
        tunnel: w8 -> [_ w338]
        tunnel: FALSE -> [_ w337]
        frame False {
        }
        frame True {
          n225 = call-poly <vilib>:"Write To Spreadsheet File.vi"("transpose? (no:F)"=w337, "1D data"=w338, "file path (dialog if empty)"=w339) -> ()  [unwired: 5 in, 1 out]
        }
      }
      n226 = case shown="True" "采集开关" {
        tunnel: w12 -> [_ w342]
        tunnel: w11 -> [_ w341]
        tunnel: FALSE -> [_ w340]
        frame False {
        }
        frame True {
          n227 = call-poly <vilib>:"Write To Spreadsheet File.vi"("transpose? (no:F)"=w340, "1D data"=w341, "file path (dialog if empty)"=w342) -> ()  [unwired: 5 in, 1 out]
        }
      }
      n228 = case shown="True" "采集开关" {
        tunnel: w21 -> [_ w351]
        tunnel: w20 -> [_ w350]
        tunnel: FALSE -> [_ w349]
        frame False {
        }
        frame True {
          n229 = call-poly <vilib>:"Write To Spreadsheet File.vi"("transpose? (no:F)"=w349, "1D data"=w350, "file path (dialog if empty)"=w351) -> ()  [unwired: 5 in, 1 out]
        }
      }
      n230 = case shown="True" "采集开关" {
        tunnel: w43 -> [_ w375]
        tunnel: w44 -> [_ w374]
        tunnel: FALSE -> [_ w373]
        frame False {
        }
        frame True {
          n231 = call-poly <vilib>:"Write To Spreadsheet File.vi"("transpose? (no:F)"=w373, "1D data"=w374, "file path (dialog if empty)"=w375) -> ()  [unwired: 5 in, 1 out]
        }
      }
      n232 = case shown="True" "采集开关" {
        tunnel: w27 -> [_ w357]
        tunnel: w26 -> [_ w356]
        tunnel: FALSE -> [_ w355]
        frame False {
        }
        frame True {
          n233 = call-poly <vilib>:"Write To Spreadsheet File.vi"("transpose? (no:F)"=w355, "1D data"=w356, "file path (dialog if empty)"=w357) -> ()  [unwired: 5 in, 1 out]
        }
      }
      n234 = case shown="True" "采集开关" {
        tunnel: w39 -> [_ w369]
        tunnel: w38 -> [_ w368]
        tunnel: FALSE -> [_ w367]
        frame False {
        }
        frame True {
          n235 = call-poly <vilib>:"Write To Spreadsheet File.vi"("transpose? (no:F)"=w367, "1D data"=w368, "file path (dialog if empty)"=w369) -> ()  [unwired: 5 in, 1 out]
        }
      }
      n236 = case shown="True" "采集开关" {
        tunnel: w33 -> [_ w363]
        tunnel: w32 -> [_ w362]
        tunnel: FALSE -> [_ w361]
        frame False {
        }
        frame True {
          n237 = call-poly <vilib>:"Write To Spreadsheet File.vi"("transpose? (no:F)"=w361, "1D data"=w362, "file path (dialog if empty)"=w363) -> ()  [unwired: 5 in, 1 out]
        }
      }
      n238 = case shown="True" "采集开关" {
        tunnel: w36 -> [_ w366]
        tunnel: w35 -> [_ w365]
        tunnel: FALSE -> [_ w364]
        frame False {
        }
        frame True {
          n239 = call-poly <vilib>:"Write To Spreadsheet File.vi"("transpose? (no:F)"=w364, "1D data"=w365, "file path (dialog if empty)"=w366) -> ()  [unwired: 5 in, 1 out]
        }
      }
      n240 = case shown="True" "采集开关" {
        tunnel: w15 -> [_ w345]
        tunnel: w14 -> [_ w344]
        tunnel: FALSE -> [_ w343]
        frame False {
        }
        frame True {
          n241 = call-poly <vilib>:"Write To Spreadsheet File.vi"("transpose? (no:F)"=w343, "1D data"=w344, "file path (dialog if empty)"=w345) -> ()  [unwired: 5 in, 1 out]
        }
      }
      n242 = case shown="True" "采集开关" {
        tunnel: w30 -> [_ w360]
        tunnel: w29 -> [_ w359]
        tunnel: FALSE -> [_ w358]
        frame False {
        }
        frame True {
          n243 = call-poly <vilib>:"Write To Spreadsheet File.vi"("transpose? (no:F)"=w358, "1D data"=w359, "file path (dialog if empty)"=w360) -> ()  [unwired: 5 in, 1 out]
        }
      }
      n244 = case shown="True" "采集开关" {
        tunnel: w48 -> [_ w378]
        tunnel: w47 -> [_ w377]
        tunnel: FALSE -> [_ w376]
        frame False {
        }
        frame True {
          n245 = call-poly <vilib>:"Write To Spreadsheet File.vi"("transpose? (no:F)"=w376, "1D data"=w377, "file path (dialog if empty)"=w378) -> ()  [unwired: 5 in, 1 out]
        }
      }
      n246 = case shown="True" "采集开关" {
        tunnel: w24 -> [_ w354]
        tunnel: w23 -> [_ w353]
        tunnel: FALSE -> [_ w352]
        frame False {
        }
        frame True {
          n247 = call-poly <vilib>:"Write To Spreadsheet File.vi"("transpose? (no:F)"=w352, "1D data"=w353, "file path (dialog if empty)"=w354) -> ()  [unwired: 5 in, 1 out]
        }
      }
      n248 = case shown="True" "采集开关" {
        tunnel: w42 -> [_ w372]
        tunnel: w41 -> [_ w371]
        tunnel: FALSE -> [_ w370]
        frame False {
        }
        frame True {
          n249 = call-poly <vilib>:"Write To Spreadsheet File.vi"("transpose? (no:F)"=w370, "1D data"=w371, "file path (dialog if empty)"=w372) -> ()  [unwired: 5 in, 1 out]
        }
      }
      n250 = case shown="True" "采集开关" {
        tunnel: w18 -> [_ w348]
        tunnel: w17 -> [_ w347]
        tunnel: FALSE -> [_ w346]
        frame False {
        }
        frame True {
          n251 = call-poly <vilib>:"Write To Spreadsheet File.vi"("transpose? (no:F)"=w346, "1D data"=w347, "file path (dialog if empty)"=w348) -> ()  [unwired: 5 in, 1 out]
        }
      }
      "通道数" <- w319
      "通道数 2" <- w306
      "通道数 3" <- w292
      "通道数 4" <- w278
      "通道数 5" <- w264
      "通道数 6" <- w250
      "通道数 7" <- w236
      "通道数 8" <- w222
      "通道数 9" <- w189
      "通道数 10" <- w173
      "通道数 11" <- w154
      "通道数 12" <- w138
      "通道数 13" <- w119
      "通道数 14" <- w103
      "通道数 15" <- w84
      "通道数 16" <- w68
    }
  }
